vi "Pendulum_PC.vi"() -> ()   [LabVIEW 2018]
uses:
  Model/Target.ctl
  Model/States.ctl
  ctl/state-machine.ctl
  <vilib>/Simulation/Scripting/Companion Diagram/SimConfigNode/SimParams.ctl
  <vilib>/Simulation/Scripting/Companion Diagram/SimConfigNode/_simSolvers.ctl
  <vilib>/Simulation/Implementation/Shared/SIMSCR Execution Mode.ctl
  <vilib>/Simulation/Param Hierarchy/Typedefs/SIMPH Param Control Actions.ctl
  <vilib>/Simulation/Implementation/Shared/NILVSim_ParamChanged.vi
  <vilib>/Simulation/Implementation/Shared/NILVSIM_BeginStep.vi
  <vilib>/Simulation/Implementation/Shared/NILVSim_Manager.vi
  <vilib>/Utility/error.llb/Clear Errors.vi
  <vilib>/Simulation/Implementation/Shared/NILVSim_FinalizeModel.vi
  vis/Global_val.vi
  <vilib>/Simulation/Implementation/Shared/SIM Unbundle Sim Info.vi
  <vilib>/Simulation/Implementation/Shared/NILVSim_Initialize.vi
  <vilib>/Simulation/Utility/Implementation/NILVSim Get Time and IsAcceptedStep.vi
  <vilib>/Simulation/Implementation/Shared/SIMSH Read Queue.vi
  <vilib>/Simulation/Implementation/Shared/NILVSim_GetModelError.vi
  <vilib>/Simulation/Implementation/Shared/SIM Bundle Sim Info.vi
  <vilib>/Simulation/Scripting/Companion Diagram/SimConfigNode/SimDog.xnode
  Model/Cart Pendulum Model.vi
  <vilib>/Simulation/Implementation/XNodeFramework/SimXNode/SimX.xnode
  <vilib>/Simulation/Implementation/Shared/NI_SIM_Implementation.lvlib
panel:
  in  "Tab Control":enum32{"config", "run"}(tab)=enum."run"
  in  "move_real":u16=1330
  in  "Mode":bool
  in  "move_step":dbl=0.03
  in  "Ini States":T1=[0.0, 0.0, 0.0, 0.0] format="%.4f"
  in  "Ini Target":T2={"Position"=0.0, "Invert"=TRUE} {"Position" min=-0.5 max=0.5 step=0.1 format="%.2g"}
  in  "play_type":enum16{"pendulum", "swing up"}(ring)
  out "status_now":string
  in  "display tab":enum32{"2D", "3D"}(tab)
  out "Pre Score":string
  out "Pendulum":picture
  out "Curr Score":string
  out "3D Picture":refnum<vi>(3d-picture)
  out "status_history":string
  in  "stop":bool
  out "timer":dbl(knob) scale=0.0..15.0
  in  "start":bool
  out "Seconds":dbl format="%.2f"
  out "Off Track":bool
  out "States":T1 format="%.4f"
  out "loop":i32
  in  "left":bool
  in  "right":bool
  in  "pos":dbl(slide) scale=-0.5..0.5
  in  "timeout s":u16=15
  in  "angle_limit":dbl=2.0 format="%#_13g"
  out "read_data":string
  out "connected":bool
  out "dt_daq":u32
  out "dt_tcp":u32
  out "main loop":i32
  in  "auto":bool
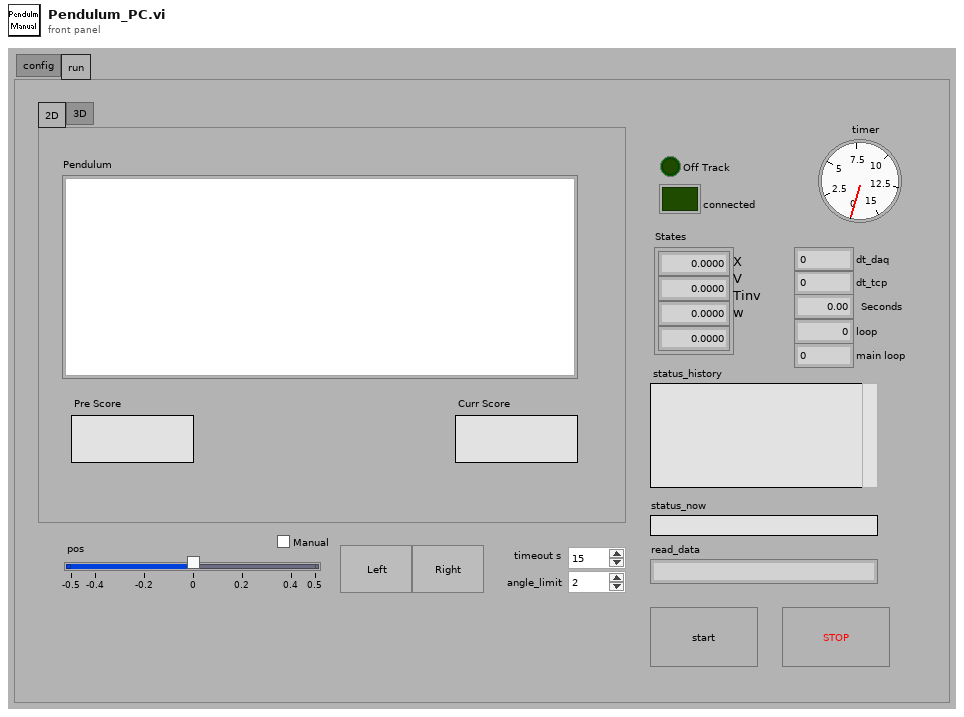
[diagram p1: front panel]
types:
  T1 = typedef "States.ctl" = dbl[]
  T2 = typedef "Target.ctl" = cluster{"Position":dbl, "Invert":bool}
  T3 = typedef "state-machine.ctl" = enum16{"wait for action", "init", "tcp_write", "tcp_read", "pause", "wait for python"}
  T4 = enum8{"Enabled", "Disabled", "Disabled and Grayed Out"}
  T5 = cluster{"connected":refnum<vi>, "start":refnum<vi>, "read_data":refnum<vi>, "Target":refnum<vi>, "play_type":refnum<vi>, "dt_daq":refnum<vi>, "dt_tcp":refnum<vi>, "timer":refnum<vi>, "States":refnum<vi>, "angle_limit":refnum<vi>, "Initial States":refnum<vi>}
  T6 = cluster{"connected":refnum<vi>, "start":refnum<vi>, "read_data":refnum<vi>, "Target":refnum<vi>, "play_type":refnum<vi>, "dt_daq":refnum<vi>, "dt_tcp":refnum<vi>, "timer":refnum<vi>, "States":refnum<vi>, "angle_limit":refnum<vi>, "Ini States":refnum<vi>}
  T7 = typedef "SIMSCR Execution Mode.ctl" = enum16{"Simulate to Completion", "Single Time-Step Simulation (Fixed Step Only)"}
  T8 = typedef "SIMPH Param Control Actions.ctl" = enum16{"get params", "set params"}
  T9 = cluster{"SIMSH Sim Time":dbl, "Integrator 3":cluster{"output":dbl[]}, "Build Array":cluster{"appended array":dbl[]}, "Index Array":cluster{"element":dbl}, "Negate 2":cluster{"-x":dbl}, "Negate":cluster{"-x":dbl}, "Sine & Cosine":cluster{"sin(x)":dbl, "cos(x)":dbl}, "Formula Node":cluster{"dx":dbl, "ddx":dbl, "dT":dbl, "ddT":dbl}}
  T10 = typedef "SimParams.ctl" = cluster{"Initial Time (s)":dbl, "Final Time (s)":dbl, "Step Size (s)":dbl, "ODE Solver":T11, "Minimum Step Size (s)":dbl, "Maximum Step Size (s)":dbl, "Relative Tolerance":dbl, "Absolute Tolerance":dbl, "Software Timing":bool, "Initial Step Size (s)":dbl, "Automatic Fixed Step Size?":bool, "Automatic Discrete Step Size?":bool, "Discrete Step Size (s)":dbl, "Calculate using Time Step":bool, "Solver Wired?":bool, "Prev.Frm.Expected End":u64, "Prev.Frm.Actual End":u64, "Prev.Frm.Finished Late?":bool, "Prev.Iter.Expected End":u64, "Prev.Iter.Actual End":u64, "Prev.Iter.Finished Late?":bool, "Expected Iteration Start":u64, "Actual Iteration Start":u64, "Expected Frame Start":u64, "Actual Frame Start":u64, "Source Name":string, "Name":string, "Period":i64, "Deadline":i64, "Offset":i64, "Start":i64, "Priority":i32, "Timeout":i32, "Processor":i32, "Mode":enum32{"No Change", "Process missed periods, maintain original phase", "Discard missed periods, maintain original phase", "Process missed periods, ignore original phase", "Discard missed periods, ignore original phase"}, "Wakeup reason":enum32{"Normal", "Aborted", "Asynchronous wakeup", "Timing source error", "Timed loop error", "Timeout"}, "Error":errorcluster, "Source Type":string, "Secondary Source Type":string, "Global End Time":u64, "Global Start Time":u64, "Full Solver Reset":bool, "Execution Mode":T7, "Nan/Inf Check":bool, "Custom Solver Library":string, "Solver Is Variable":bool, "custom solver name":string, "Signal Collection Decimation":u32}
  T11 = typedef "_simSolvers.ctl" = enum16{"Runge-Kutta 1 (Euler)", "Runge-Kutta 2", "Runge-Kutta 3", "Runge-Kutta 4", "Runge-Kutta 23 (variable)", "Runge-Kutta 45 (variable)", "BDF (variable)", "Adams-Moulton (variable)", "Rosenbrock (variable)", "Discrete States Only", "SDIRK 4 (variable)", "Radau 5 (variable)", "Radau 9 (variable)", "Radau 13 (variable)", "Radau [Variable Order] (variable)", "Gear's Method (variable)", "Linearizer", "State Query", "Trim Eval", "Custom Solver"}
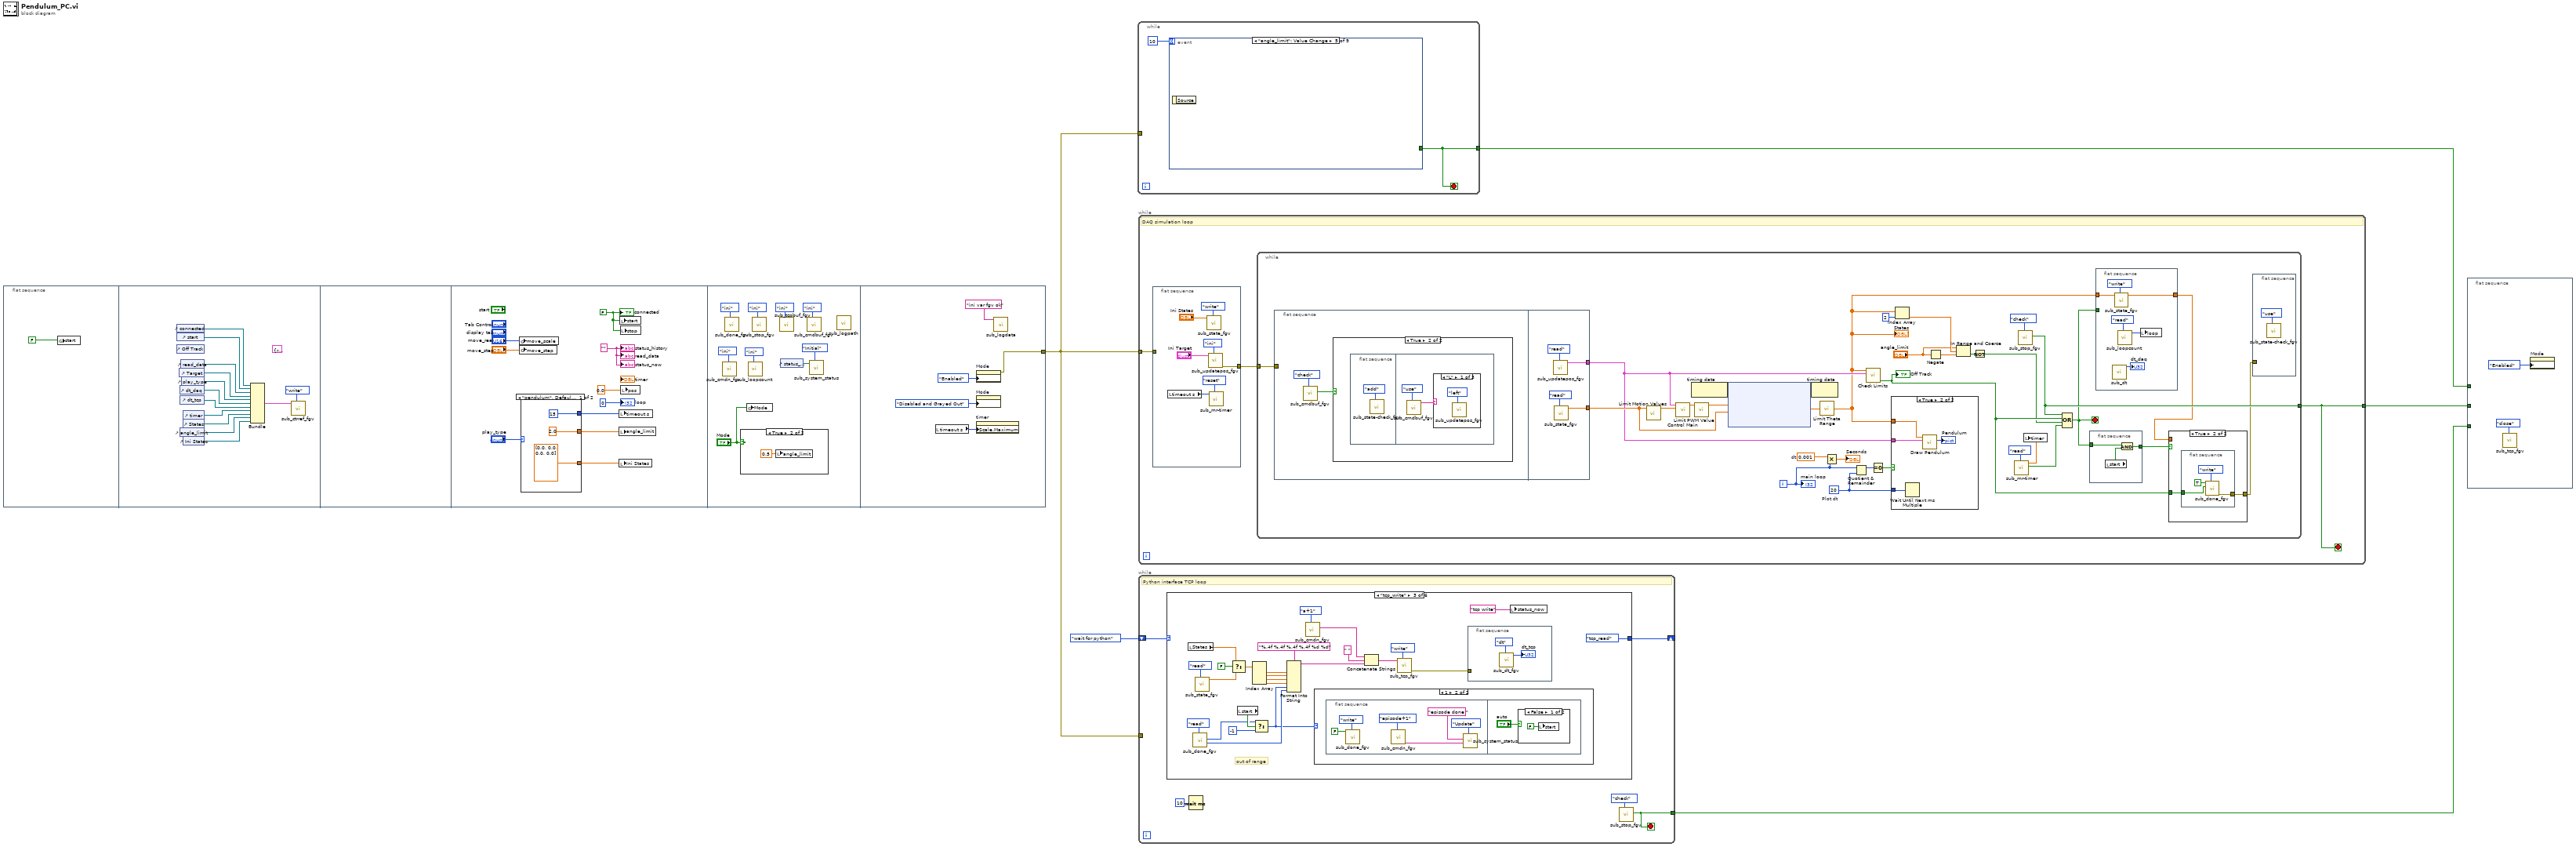
[diagram p0: block diagram]
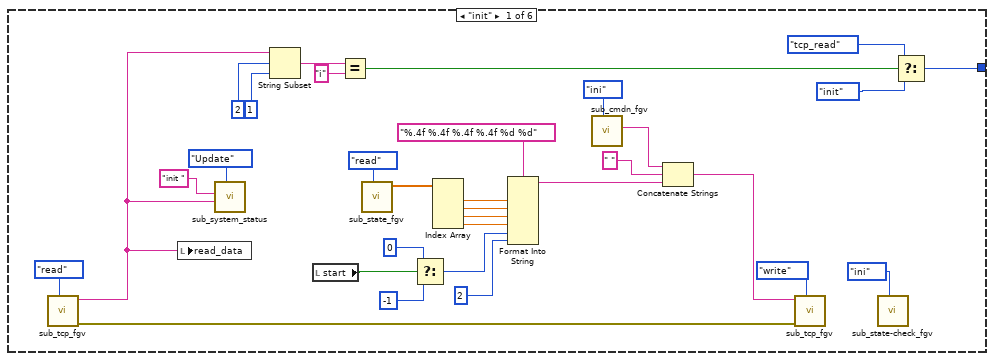
[diagram p2: hidden frame]
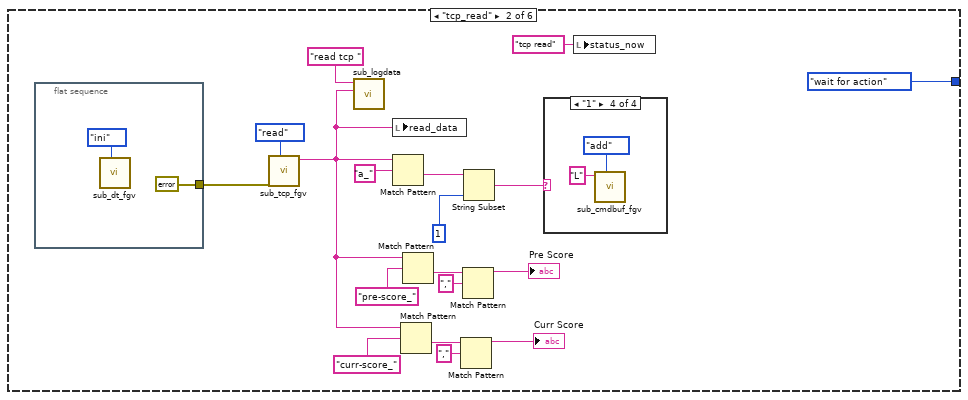
[diagram p3: hidden frame]
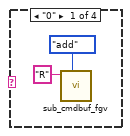
[diagram p4: hidden frame]
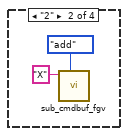
[diagram p5: hidden frame]
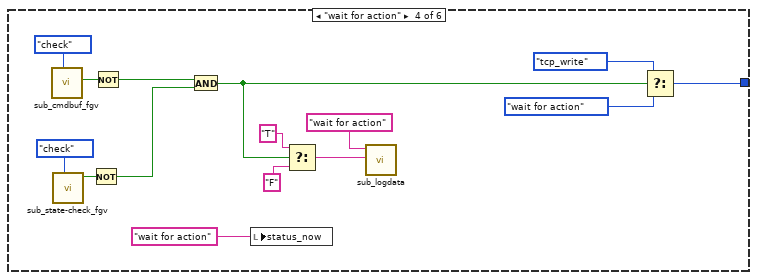
[diagram p9: hidden frame]
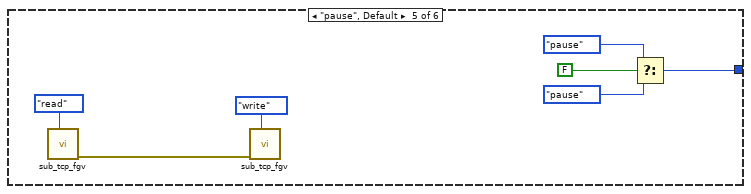
[diagram p10: hidden frame]
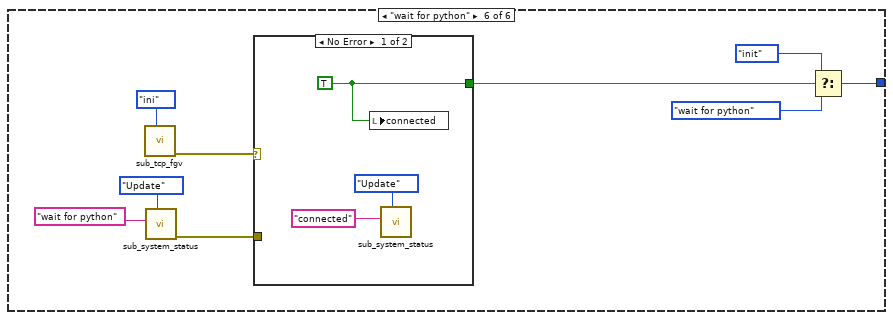
[diagram p11: hidden frame]
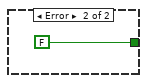
[diagram p12: hidden frame]
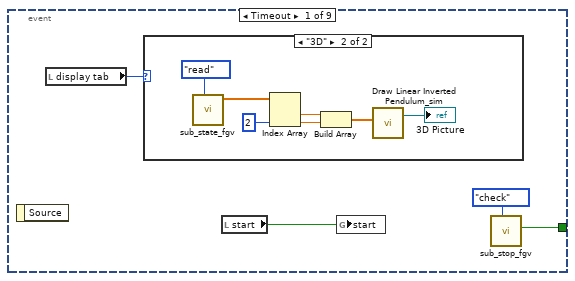
[diagram p13: hidden frame]
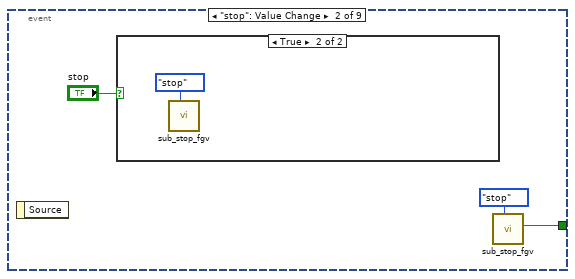
[diagram p15: hidden frame]
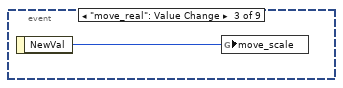
[diagram p17: hidden frame]
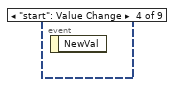
[diagram p18: hidden frame]
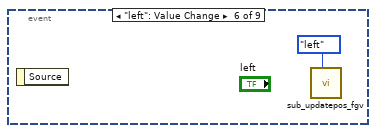
[diagram p19: hidden frame]
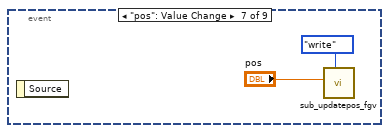
[diagram p20: hidden frame]
diagram:
  n1 = flat-sequence {
    tunnel: [w46] -> w1
    frame #0 {
      n2 = global write "Global_val.vi" "start"(FALSE ("stop")) -> ()
    }
    frame #1 {
      (unwired) T5 {"connected"=refnum, "start"=refnum, "read_data"=refnum, "Target"=refnum, "play_type"=refnum, "dt_daq"=refnum, "dt_tcp"=refnum, "timer"=refnum, "States"=refnum, "angle_limit"=refnum, "Initial States"=refnum} ("output cluster")
      n3 = control-ref of="connected"() -> (w19:refnum<vi>)
      n4 = control-ref of="start"() -> (w18:refnum<vi>)
      n5 = control-ref of="Off Track"() -> ()  [unwired: 1 out]
      n6 = control-ref of="Target"() -> (w12:refnum<vi>)
      n7 = control-ref of="dt_daq"() -> (w11:refnum<vi>)
      n8 = control-ref of="dt_tcp"() -> (w8:refnum<vi>)
      n9 = control-ref of="angle_limit"() -> (w14:refnum<vi>)
      n10 = control-ref of="read_data"() -> (w17:refnum<vi>)
      n11 = control-ref of="play_type"() -> (w15:refnum<vi>)
      n12 = control-ref of="timer"() -> (w9:refnum<vi>)
      n13 = control-ref of="States"() -> (w10:refnum<vi>)
      n14 = control-ref of="Ini States"() -> (w13:refnum<vi>)
      n15 = Bundle("connected"=w19, "start"=w18, "read_data"=w17, "Target"=w12, "play_type"=w15, "dt_daq"=w11, "dt_tcp"=w8, "timer"=w9, "States"=w10, "angle_limit"=w14, "Ini States"=w13) -> (w7:T6)  [unwired: 1 in]
      n16 = call "sub_ctrref_fgv.vi"("cmd"=enum16{"write", "read"}."write", "ctr_in"=w7) -> ()  [unwired: 9 in, 1 out]
    }
    frame #2 {
    }
    frame #3 {
      w20 = "" ("status")
      w21 = FALSE ("ini")
      n17 = global write "Global_val.vi" "move_scale"("move_real") -> ()
      n18 = global write "Global_val.vi" "move_step"("move_step") -> ()
      n19 = case shown="\"pendulum\", Default" "play_type" {
        tunnel: [T1 [0.0, 0.0, 0.0, 0.0] ("Initial States") T1 [0.0, 0.0, 3.14, 0.0] ("Initial States")] -> w27
        tunnel: [2.0 ("pos_limit") 4.0 ("pos_limit")] -> w26
        tunnel: [u16 15 ("timeout s") u16 25 ("timeout s")] -> w25
        frame "pendulum", Default {
        }
        frame "swing up" {
        }
      }
      n20 = local write "timeout s"(w25) -> ()
      n21 = local write "angle_limit"(w26) -> ()
      n22 = local write "Ini States"(w27) -> ()
      n23 = local write "start"(w21) -> ()
      n24 = local write "stop"(w21) -> ()
      n25 = local write "pos"(0.0 ("pos")) -> ()
      "status_history" <- w20
      "connected" <- w21
      "read_data" <- w20
      "loop" <- 0 ("loop")
      "status_now" <- w20
    }
    frame #4 {
      n26 = call "sub_cmdn_fgv.vi"("cmd"=enum16{"ini", "a+1", "episode+1", "read"}."ini") -> ()  [unwired: 7 in, 4 out]
      n27 = call "sub_done_fgv.vi"("cmd"=enum16{"ini", "write", "read"}."ini") -> ()  [unwired: 8 in, 3 out]
      n28 = case shown="True" "Mode" {
        frame False {
        }
        frame True {
          n29 = local write "angle_limit"(0.5 ("angle_limit")) -> ()
        }
      }
      n30 = global write "Global_val.vi" "Mode"("Mode") -> ()
      n31 = call "sub_loopcount.vi"("cmd"=enum16{"ini", "count 1", "read"}."ini") -> ()  [unwired: 10 in, 1 out]
      n32 = call "sub_stop_fgv.vi"("cmd"=enum16{"ini", "check", "stop"}."ini") -> ()  [unwired: 10 in, 1 out]
      n33 = call "sub_tcpbuf_fgv.vi"("cmd"=enum16{"ini", "add", "use", "check"}."ini") -> ()  [unwired: 8 in, 3 out]
      n34 = control-ref of="status_history"() -> (w42:refnum<vi>)
      n35 = call "sub_cmdbuf_fgv.vi"("cmd"=enum16{"ini", "add", "use", "check"}."ini") -> ()  [unwired: 9 in, 2 out]
      n36 = call "sub_system_status.vi"("Mode"=enum16{"Initial", "Update", "Clear"}."Initial", "System Log"=w42) -> ()  [unwired: 9 in, 1 out]
      n37 = call "sub_logpath.vi"() -> ()  [unwired: 11 in, 1 out]
    }
    frame #5 {
      n38 = local read "timeout s"() -> (w49:u16)
      n39 = property on="Mode" class="Bool (strict)"("DisabledEnum"=T4."Enabled" ("Disabled")) -> (error out=w46:errorcluster)  [unwired: 2 in, 1 out]
      n40 = property on="Mode" class="Bool (strict)"("DisabledEnum"=T4."Disabled and Grayed Out" ("Disabled")) -> ()  [unwired: 2 in, 2 out]
      n41 = property on="timer" class="Knob (strict)"("Scale.Maximum"=w49) -> ()  [unwired: 2 in, 2 out]
      n42 = call "sub_logdata.vi"("Title"="ini var fgv ok") -> ()  [unwired: 10 in, 1 out]
    }
  }
  n43 = while {
    tunnel: w1 -> [_]
    tunnel: [w52] -> w4
    stop <- w52 stop-if-true
    n44 = event shown="[4] \"angle_limit\": Value Change" {
      selector: _ -> [_ _ _ _ _ _ _ _ _]
      dyn-events: _ -> [_ _ _ _ _ _ _ _ _]
      timeout: 10 -> [_ _ _ _ _ _ _ _ _]
      tunnel: [w55 w65 _ _ _ _ _ _ _] -> w52
      event Timeout {
        n45 = event-data() -> ()  [unwired: 1 in, 1 out]
        n46 = local read "display tab"() -> (w54:enum32{"2D", "3D"})
        n47 = case shown="\"3D\"" w54 {
          frame "2D", Default {
          }
          frame "3D" {
            n48 = call "sub_state_fgv.vi"("cmd"=enum16{"read", "write"}."read") -> ("state_out"=w59:dbl[])  [unwired: 10 in]
            n49 = Index Array(array=w59, index #2=2 ("index")) -> (element #1=w60:dbl, element #2=w61:dbl)  [unwired: 1 in]
            n50 = Build Array(w60, w61) -> (w62:dbl[])
            n51 = call "Draw Linear Inverted Pendulum_sim.vi"("Linear Pos and Angle"=w62) -> ("Scene.New Object"=→"3D Picture":refnum<vi>)  [unwired: 4 in, 1 out]
          }
        }
        n52 = local read "start"() -> (w53:bool)
        n53 = global write "Global_val.vi" "start"(w53) -> ()
        n54 = call "sub_stop_fgv.vi"("cmd"=enum16{"ini", "check", "stop"}."check") -> ("status"=w55:bool)  [unwired: 10 in]
      }
      event "stop": Value Change {
        n55 = event-data() -> ()  [unwired: 1 in, 1 out]
        n56 = case shown="True" "stop" {
          frame False {
          }
          frame True {
            n57 = call "sub_stop_fgv.vi"("cmd"=enum16{"ini", "check", "stop"}."stop") -> ()  [unwired: 10 in, 1 out]
          }
        }
        n58 = call "sub_stop_fgv.vi"("cmd"=enum16{"ini", "check", "stop"}."stop") -> ("status"=w65:bool)  [unwired: 10 in]
      }
      event "move_real": Value Change {
        n59 = event-data() -> ("NewVal"=w68:u16)  [unwired: 1 in]
        n60 = global write "Global_val.vi" "move_scale"(w68) -> ()
      }
      event "start": Value Change {
        n61 = event-data() -> ()  [unwired: 1 in, 1 out]
      }
      event "angle_limit": Value Change {
        n62 = event-data() -> ()  [unwired: 1 in, 1 out]
      }
      event "left": Value Change {
        n63 = event-data() -> ()  [unwired: 1 in, 1 out]
        n64 = call "sub_updatepos_fgv.vi"("cmd"=enum16{"left", "right", "ini", "read", "write"}."left") -> ()  [unwired: 9 in, 2 out]
      }
      event "pos": Value Change {
        n65 = event-data() -> ()  [unwired: 1 in, 1 out]
        n66 = call "sub_updatepos_fgv.vi"("cmd"=enum16{"left", "right", "ini", "read", "write"}."write", "pos"="pos") -> ()  [unwired: 8 in, 2 out]
      }
      event "right": Value Change {
        n67 = event-data() -> ()  [unwired: 1 in, 1 out]
        n68 = call "sub_updatepos_fgv.vi"("cmd"=enum16{"left", "right", "ini", "read", "write"}."right") -> ()  [unwired: 9 in, 2 out]
      }
      event "timeout s": Value Change {
        n69 = event-data() -> ()  [unwired: 1 in, 1 out]
        n70 = property on="timer" class="Knob (strict)"("Scale.Maximum"="timeout s") -> ()  [unwired: 2 in, 2 out]
        n71 = call "sub_mr-timer.vi"("cmd"=enum16{"reset", "read"}."reset", "limit s"="timeout s") -> ()  [unwired: 8 in, 2 out]
      }
    }
  }
  n72 = while {
    tunnel: w1 -> [w75]
    tunnel: [w77] -> w3
    stop <- w77 stop-if-true
    # "DAQ simulation loop"
    n73 = flat-sequence {
      tunnel: [w78] -> w76
      tunnel: w75 -> [_]
      frame #0 {
        n74 = local read "timeout s"() -> (w79:u16)
        n75 = call "sub_state_fgv.vi"("cmd"=enum16{"read", "write"}."write", "Initial States"="Ini States") -> ()  [unwired: 9 in, 1 out]
        n76 = call "sub_updatepos_fgv.vi"("cmd"=enum16{"left", "right", "ini", "read", "write"}."ini", "Target"="Ini Target") -> ("error out"=w78:errorcluster)  [unwired: 8 in, 1 out]
        n77 = call "sub_mr-timer.vi"("cmd"=enum16{"reset", "read"}."reset", "limit s"=w79) -> ()  [unwired: 8 in, 2 out]
      }
    }
    n78 = while {
      tunnel: [w102] -> w77
      tunnel: w76 -> [w87]
      i -> [w98]
      stop <- w97 stop-if-true
      w88 = u32 20  # Plot dt
      w104 = 0.001  # dt
      n79 = flat-sequence {
        tunnel: w87 -> [_]
        tunnel: [w379] -> w103
        tunnel: [w377] -> w114
        frame #0 {
          n80 = call "sub_cmdbuf_fgv.vi"("cmd"=enum16{"ini", "add", "use", "check"}."check") -> ("data"=w370:bool)  [unwired: 9 in, 1 out]
          n81 = case shown="True" w370 {
            frame False {
            }
            frame True {
              n82 = flat-sequence {
                frame #0 {
                  n83 = call "sub_state-check_fgv.vi"("cmd"=enum16{"ini", "add", "use", "check"}."add") -> ()  [unwired: 8 in, 3 out]
                }
                frame #1 {
                  n84 = call "sub_cmdbuf_fgv.vi"("cmd"=enum16{"ini", "add", "use", "check"}."use") -> ("element"=w373:string)  [unwired: 9 in, 1 out]
                  n85 = case shown="\"L\"" w373 {
                    frame "L" {
                      n86 = call "sub_updatepos_fgv.vi"("cmd"=enum16{"left", "right", "ini", "read", "write"}."left") -> ()  [unwired: 9 in, 2 out]
                    }
                    frame Default {
                    }
                    frame "R" {
                      n87 = call "sub_updatepos_fgv.vi"("cmd"=enum16{"left", "right", "ini", "read", "write"}."right") -> ()  [unwired: 9 in, 2 out]
                    }
                  }
                }
              }
            }
          }
        }
        frame #1 {
          n88 = call "sub_updatepos_fgv.vi"("cmd"=enum16{"left", "right", "ini", "read", "write"}."read") -> ("Target_out"=w379:T2)  [unwired: 9 in, 1 out]
          n89 = call "sub_state_fgv.vi"("cmd"=enum16{"read", "write"}."read") -> ("state_out"=w377:dbl[])  [unwired: 10 in]
        }
      }
      n90 = call "Limit Motion Values.vi"("States In"=w114) -> ("States Out"=w93:T1)  [unwired: 10 in]
      n91 = call "Control Main.vi"("States"=w93, "Target"=w103) -> ("PWM"=w92:dbl)  [unwired: 9 in]
      n92 = node-c288() -> (w95:variant)  [unwired: 1 in]
      n93 = call "Limit PWM Value.vi"("PWM In"=w92) -> ("PWM Out"=w91:dbl)  [unwired: 10 in]
      n94 = node-c254 ("Control & Simulation Loop 2")(w95, w91, w114) -> (w94:variant, w90:dbl[])
      n95 = node-c288(w94) -> ()  [unwired: 1 out]
      n96 = call "Limit Theta Range.vi"("States In"=w90) -> ("States Out"=w89:T1)
      "States" <- w89
      n97 = Multiply(x=w104, y=w98) -> (x*y=→"Seconds":dbl)
      n98 = Quotient & Remainder(x=w98, y=w88) -> (x-y*floor(x/y)=w107:u32)  [unwired: 1 out]
      n99 = call "Check Limits.vi"("Target"=w103, "States"=w89) -> ("Off Track"=w101:bool)  [unwired: 3 in, 3 out]
      "Off Track" <- w101
      n100 = Equal To 0?(x=w107) -> (x = 0?=w106:bool)
      n101 = case shown="True" w106 {
        tunnel: w89 -> [_ w354]
        tunnel: w103 -> [_ w356]
        tunnel: w88 -> [_ w355]
        frame False {
        }
        frame True {
          n102 = Wait Until Next ms Multiple(millisecond multiple=w355) -> ()  [unwired: 1 out]
          n103 = call "Draw Pendulum.vi"("Target"=w356, "States In"=w354) -> ("Picture"=→"Pendulum":picture)  [unwired: 1 in, 8 out]
        }
      }
      n104 = Index Array(array=w89, index=2) -> (element=w111:dbl)
      n105 = Negate(x="angle_limit") -> (-x=w110:dbl)
      n106 = In Range and Coerce(upper limit="angle_limit", x=w111, lower limit=w110) -> (In Range?=w109:bool)  [unwired: 1 out]
      n107 = Not(x=w109) -> (.not. x?=w100:bool)
      n108 = call "sub_mr-timer.vi"("cmd"=enum16{"reset", "read"}."read") -> ("timeout"=w99:bool, "time"=w113:dbl)  [unwired: 9 in]
      n109 = call "sub_stop_fgv.vi"("cmd"=enum16{"ini", "check", "stop"}."check") -> ("status"=w102:bool)  [unwired: 10 in]
      n110 = local write "timer"(w113) -> ()
      n111 = Compound Arithmetic op=OR(w102, w101, w100, w99) -> (w97:bool)
      n112 = flat-sequence {
        tunnel: w97 -> [w352]
        tunnel: [w351] -> w96
        frame #0 {
          n113 = local read "start"() -> (w353:bool)
          n114 = And(x=w352, y=w353) -> (x .and. y?=w351:bool)
        }
      }
      n115 = flat-sequence {
        tunnel: w97 -> [_]
        tunnel: w89 -> [w359]
        tunnel: [w358] -> w86
        frame #0 {
          n116 = call "sub_dt.vi"() -> ("dt"=→"dt_daq":u32)  [unwired: 11 in]
          n117 = call "sub_state_fgv.vi"("cmd"=enum16{"read", "write"}."write", "Initial States"=w359) -> ("state_out"=w358:dbl[])  [unwired: 9 in]
          n118 = call "sub_loopcount.vi"("cmd"=enum16{"ini", "count 1", "read"}."read") -> ("countn"=w362:u32)  [unwired: 10 in]
          n119 = local write "loop"(w362) -> ()
        }
      }
      n120 = case shown="True" w96 {
        tunnel: w101 -> [_ w365]
        tunnel: [_ w364] -> w85
        tunnel: w86 -> [_ _]
        frame False {
        }
        frame True {
          n121 = flat-sequence {
            tunnel: w365 -> [w367]
            tunnel: [w366] -> w364
            frame #0 {
              n122 = call "sub_done_fgv.vi"("cmd"=enum16{"ini", "write", "read"}."write", "off_track"=w367, "input"=TRUE) -> ("error out"=w366:errorcluster)  [unwired: 6 in, 2 out]
            }
          }
        }
      }
      n123 = flat-sequence {
        tunnel: w85 -> [_]
        frame #0 {
          n124 = call "sub_state-check_fgv.vi"("cmd"=enum16{"ini", "add", "use", "check"}."use") -> ()  [unwired: 8 in, 3 out]
        }
      }
      "main loop" <- w98
    }
  }
  n125 = while {
    tunnel: w1 -> [_]
    shift-right: [w381] -> _
    shift-left: state-machine."wait for python" ("state") -> [w382]
    tunnel: [w383] -> w2
    stop <- w383 stop-if-true
    # "Python interface TCP loop"
    n126 = case shown="\"tcp_write\"" w382 {
      tunnel: [w417 state-machine."wait for action" ("state") state-machine."tcp_read" ("f") w491 w498 w505] -> w381
      frame "init" {
        n127 = call "sub_tcp_fgv.vi"("cmd"=enum16{"ini", "read", "write", "close"}."read") -> ("error out"=w391:errorcluster, "read_data"=w388:string)  [unwired: 8 in, 1 out]
        n128 = local write "read_data"(w388) -> ()
        n129 = call "sub_system_status.vi"("Mode"=enum16{"Initial", "Update", "Clear"}."Update", "content"=w388, "title"="init " ("String in")) -> ()  [unwired: 8 in, 1 out]
        n130 = String Subset(string=w388, offset (0)=2, length (rest)=1 ("length (rest)")) -> (substring=w411:string)
        n131 = local read "start"() -> (w389:bool)
        n132 = Equal?(x=w411, y="i") -> (x = y?=w392:bool)
        n133 = call "sub_state_fgv.vi"("cmd"=enum16{"read", "write"}."read") -> ("state_out"=w409:dbl[])  [unwired: 10 in]
        n134 = Select(t=i8 0, s=w389, f=i8 -1) -> (s? t:f=w403:i8)
        n135 = Index Array(array=w409) -> (element #1=w408:dbl, element #2=w407:dbl, element #3=w406:dbl, element #4=w405:dbl)  [unwired: 4 in]
        n136 = Format Into String(format string="%.4f %.4f %.4f %.4f %d %d" ("포맷 문자열"), w408, w407, w406, w405, w403, i8 2 ("입력 6")) -> (resulting string=w404:string)  [unwired: 2 in, 1 out]
        n137 = call "sub_cmdn_fgv.vi"("cmd"=enum16{"ini", "a+1", "episode+1", "read"}."ini") -> ("action_str"=w395:string)  [unwired: 7 in, 3 out]
        n138 = Concatenate Strings(w395, " " ("구분 문자 (탭)"), w404) -> (w387:string)
        n139 = call "sub_tcp_fgv.vi"("cmd"=enum16{"ini", "read", "write", "close"}."write", "error in (no error)"=w391, "write_data"=w387) -> ()  [unwired: 6 in, 3 out]
        n140 = call "sub_state-check_fgv.vi"("cmd"=enum16{"ini", "add", "use", "check"}."ini") -> ()  [unwired: 8 in, 3 out]
        n141 = Select(t=state-machine."tcp_read", s=w392, f=state-machine."init" ("state")) -> (s? t:f=w417:T3)
      }
      frame "tcp_read" {
        n142 = flat-sequence {
          tunnel: [errorcluster {"status"=FALSE, "code"=0, "source"=""} ("error out")] -> w430
          frame #0 {
            n143 = call "sub_dt_fgv.vi"("cmd"=enum16{"ini", "dt"}."ini") -> ()  [unwired: 10 in, 1 out]
          }
        }
        n144 = call "sub_tcp_fgv.vi"("cmd"=enum16{"ini", "read", "write", "close"}."read", "error in (no error)"=w430) -> ("read_data"=w419:string)  [unwired: 7 in, 2 out]
        n145 = call "sub_logdata.vi"("data_str"=w419, "Title"="read tcp ") -> ()  [unwired: 9 in, 1 out]
        n146 = local write "read_data"(w419) -> ()
        n147 = Match Pattern(string=w419, regular expression="a_") -> (after substring=w433:string)  [unwired: 1 in, 3 out]
        n148 = Match Pattern(string=w419, regular expression="curr-score_") -> (after substring=w421:string)  [unwired: 1 in, 3 out]
        n149 = Match Pattern(string=w419, regular expression="pre-score_") -> (after substring=w425:string)  [unwired: 1 in, 3 out]
        n150 = Match Pattern(string=w421, regular expression=",") -> (before substring=→"Curr Score":string)  [unwired: 1 in, 3 out]
        n151 = Match Pattern(string=w425, regular expression=",") -> (before substring=→"Pre Score":string)  [unwired: 1 in, 3 out]
        n152 = String Subset(string=w433, length (rest)=1 ("length (rest)")) -> (substring=w427:string)  [unwired: 1 in]
        n153 = case shown="\"1\"" w427 {
          frame "0" {
            n154 = call "sub_cmdbuf_fgv.vi"(7:"cmd"=enum16{"ini", "add", "use", "check"}."add" ("cmd"), 11:"cmd"="R" ("cmd")) -> ()  [unwired: 8 in, 2 out]
          }
          frame "2" {
            n155 = call "sub_cmdbuf_fgv.vi"(7:"cmd"=enum16{"ini", "add", "use", "check"}."add" ("cmd"), 11:"cmd"="X" ("cmd")) -> ()  [unwired: 8 in, 2 out]
          }
          frame "-1000", Default {
            # "not define"
          }
          frame "1" {
            n156 = call "sub_cmdbuf_fgv.vi"(7:"cmd"=enum16{"ini", "add", "use", "check"}."add" ("cmd"), 11:"cmd"="L" ("cmd")) -> ()  [unwired: 8 in, 2 out]
          }
        }
        n157 = local write "status_now"("tcp read" ("status_now")) -> ()
      }
      frame "tcp_write" {
        # "out of range"
        n158 = local read "States"() -> (w447:T1)
        n159 = call "sub_done_fgv.vi"("cmd"=enum16{"ini", "write", "read"}."read") -> ("range_val"=w457:i32, "done_val"=w452:i32)  [unwired: 8 in, 1 out]
        n160 = call "sub_state_fgv.vi"("cmd"=enum16{"read", "write"}."read") -> ("state_out"=w446:dbl[])  [unwired: 10 in]
        n161 = Select(t=w447, s=FALSE, f=w446) -> (s? t:f=w445:T1)
        n162 = local read "start"() -> (w453:bool)
        n163 = Index Array(array=w445) -> (element #1=w467:dbl, element #2=w466:dbl, element #3=w465:dbl, element #4=w464:dbl)  [unwired: 4 in]
        n164 = Select(t=w452, s=w453, f=-1) -> (s? t:f=w450:i32)
        n165 = Format Into String(format string="%.4f %.4f %.4f %.4f %d %d" ("포맷 문자열"), w467, w466, w465, w464, w450, w457) -> (resulting string=w463:string)  [unwired: 2 in, 1 out]
        n166 = call "sub_cmdn_fgv.vi"("cmd"=enum16{"ini", "a+1", "episode+1", "read"}."a+1") -> ("action_str"=w460:string)  [unwired: 7 in, 3 out]
        n167 = case shown="1" w450 {
          frame 0, Default {
          }
          frame 1 {
            n168 = flat-sequence {
              frame #0 {
                n169 = call "sub_done_fgv.vi"("cmd"=enum16{"ini", "write", "read"}."write", "input"=FALSE) -> ()  [unwired: 7 in, 3 out]
                n170 = call "sub_cmdn_fgv.vi"("cmd"=enum16{"ini", "a+1", "episode+1", "read"}."episode+1") -> ("episode_str"=w473:string)  [unwired: 7 in, 3 out]
                n171 = call "sub_system_status.vi"("Mode"=enum16{"Initial", "Update", "Clear"}."Update", "content"=w473, "title"="episode done ") -> ()  [unwired: 8 in, 1 out]
              }
              frame #1 {
                n172 = case shown="False" "auto" {
                  frame False {
                    n173 = local write "start"(FALSE ("start")) -> ()
                  }
                  frame True {
                  }
                }
              }
            }
          }
        }
        n174 = Concatenate Strings(w460, " " ("구분 문자 (탭)"), w463) -> (w454:string)
        n175 = call "sub_tcp_fgv.vi"("cmd"=enum16{"ini", "read", "write", "close"}."write", "write_data"=w454) -> ("error out"=w456:errorcluster)  [unwired: 7 in, 2 out]
        n176 = flat-sequence {
          tunnel: w456 -> [_]
          frame #0 {
            n177 = call "sub_dt_fgv.vi"("cmd"=enum16{"ini", "dt"}."dt") -> ("dt"=→"dt_tcp":u32)  [unwired: 10 in]
          }
        }
        n178 = local write "status_now"("tcp write" ("status_now")) -> ()
      }
      frame "wait for action" {
        n179 = call "sub_cmdbuf_fgv.vi"("cmd"=enum16{"ini", "add", "use", "check"}."check") -> ("data"=w489:bool)  [unwired: 9 in, 1 out]
        n180 = call "sub_state-check_fgv.vi"("cmd"=enum16{"ini", "add", "use", "check"}."check") -> ("data"=w479:bool)  [unwired: 8 in, 2 out]
        n181 = Not(x=w479) -> (.not. x?=w487:bool)
        n182 = Not(x=w489) -> (.not. x?=w488:bool)
        n183 = And(x=w488, y=w487) -> (x .and. y?=w484:bool)
        n184 = local write "status_now"("wait for action" ("status_now")) -> ()
        n185 = Select(t="T" ("status_now"), s=w484, f="F" ("status_now")) -> (s? t:f=w482:string)
        n186 = call "sub_logdata.vi"("data_str"=w482, "Title"="wait for action") -> ()  [unwired: 9 in, 1 out]
        n187 = Select(t=state-machine."tcp_write" ("state"), s=w484, f=state-machine."wait for action") -> (s? t:f=w491:T3)
      }
      frame "pause", Default {
        n188 = call "sub_tcp_fgv.vi"("cmd"=enum16{"ini", "read", "write", "close"}."read") -> ("error out"=w495:errorcluster)  [unwired: 8 in, 2 out]
        n189 = call "sub_tcp_fgv.vi"("cmd"=enum16{"ini", "read", "write", "close"}."write", "error in (no error)"=w495) -> ()  [unwired: 7 in, 3 out]
        n190 = Select(t=state-machine."pause" ("f"), s=FALSE, f=state-machine."pause") -> (s? t:f=w498:T3)
      }
      frame "wait for python" {
        n191 = call "sub_tcp_fgv.vi"("cmd"=enum16{"ini", "read", "write", "close"}."ini") -> ("error out"=w506:errorcluster)  [unwired: 8 in, 2 out]
        n192 = call "sub_system_status.vi"("Mode"=enum16{"Initial", "Update", "Clear"}."Update", "title"="wait for python" ("String in")) -> ("error out"=w501:errorcluster)  [unwired: 9 in]
        n193 = case shown="No Error" w506 {
          tunnel: [w510 FALSE ("s")] -> w504
          tunnel: w501 -> [_ _]
          frame No Error {
            w510 = TRUE ("s")
            n194 = local write "connected"(w510) -> ()
            n195 = call "sub_system_status.vi"("Mode"=enum16{"Initial", "Update", "Clear"}."Update", "title"="connected" ("String in")) -> ()  [unwired: 9 in, 1 out]
          }
          frame Error {
          }
        }
        n196 = Select(t=state-machine."init" ("f"), s=w504, f=state-machine."wait for python") -> (s? t:f=w505:T3)
      }
    }
    n197 = Wait (ms)(milliseconds to wait=u32 10) -> ()  [unwired: 1 out]
    n198 = call "sub_stop_fgv.vi"("cmd"=enum16{"ini", "check", "stop"}."check") -> ("status"=w383:bool)  [unwired: 10 in]
  }
  n199 = flat-sequence {
    tunnel: w4 -> [_]
    tunnel: w3 -> [_]
    tunnel: w2 -> [_]
    frame #0 {
      n200 = call "sub_tcp_fgv.vi"("cmd"=enum16{"ini", "read", "write", "close"}."close") -> ()  [unwired: 8 in, 3 out]
      n201 = property on="Mode" class="Bool (strict)"("DisabledEnum"=T4."Enabled" ("Disabled")) -> ()  [unwired: 2 in, 2 out]
    }
  }
